vi "CT_CapVoltCamBinning.vi"(2 "Bin Size Reduction":i32, 3 "Center Spacing Y":dbl, 4 "Center Spacing X":dbl, 5 "Boundry Pixel Array":T1(array[cluster])=[{"Location Label"="Top  Left", "X Pixel"=0, "Y pixel"=0}, {"Location Label"="Top Right", "X Pixel"=0, "Y pixel"=0}, {"Location Label"="Bottom Right", "X Pixel"=0, "Y pixel"=0}, {"Location Label"="Bottom Left", "X Pixel"=0, "Y pixel"=0}]) -> (0 "Bin Center Array":cluster{"X":i32, "Y":i32}[][](array[cluster]), 1 "Fiber Bin Array":u32[][](array[numeric]))   [LabVIEW 2016]
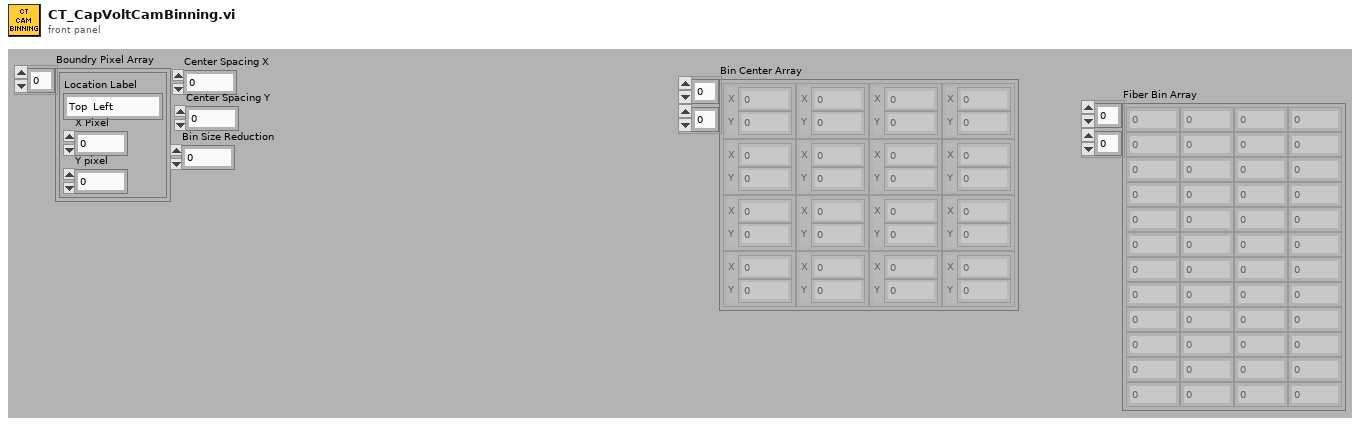
[diagram p1: front panel]
types:
  T1 = cluster{"Location Label":string, "X Pixel":i32, "Y pixel":i32}[]
  T2 = cluster{"Location Label":string, "X Pixel":i32, "Y pixel":i32}
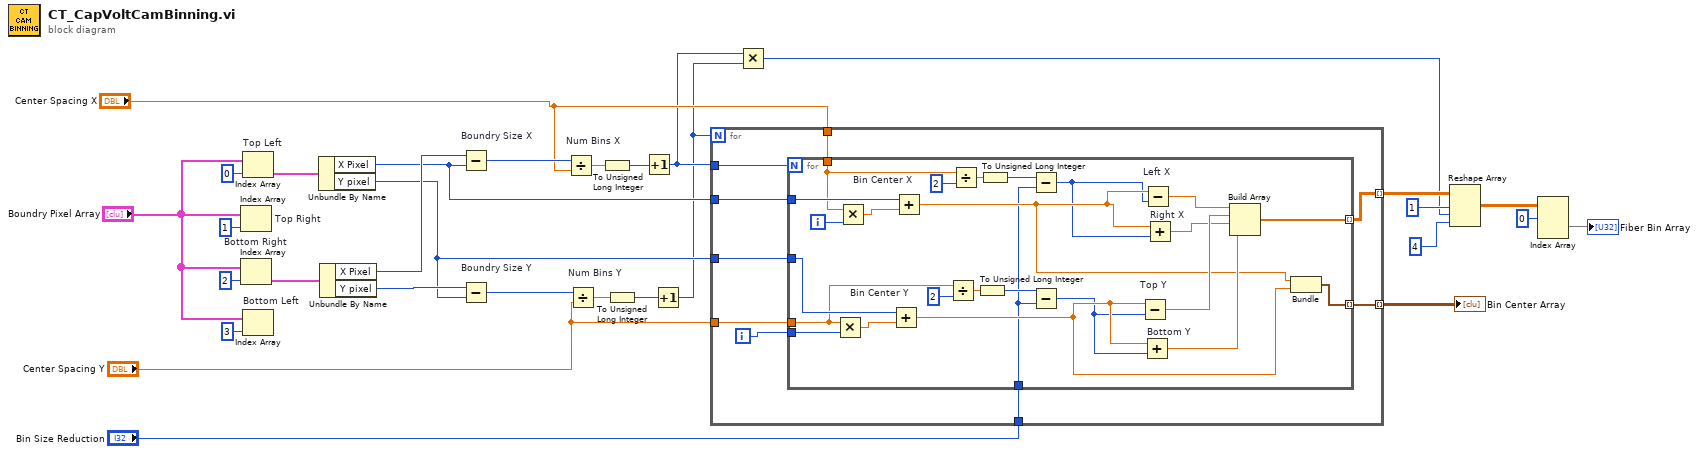
[diagram p0: block diagram]
diagram:
  n1 = Index Array "Top Right"(array="Boundry Pixel Array", index=1) -> ()  [unwired: 1 out]
  n2 = Index Array "Bottom Right"(array="Boundry Pixel Array", index=2) -> (element=w24:T2)
  n3 = Index Array "Top Left"(array="Boundry Pixel Array", index=0) -> (element=w25:T2)
  n4 = Index Array "Bottom Left"(array="Boundry Pixel Array", index=3) -> ()  [unwired: 1 out]
  n5 = Unbundle By Name(w25) -> ("X Pixel"=w17:i32, "Y pixel"=w15:i32)
  n6 = Unbundle By Name(w24) -> ("X Pixel"=w23:i32, "Y pixel"=w22:i32)
  n7 = Subtract "Boundry Size X"(x=w23, y=w17) -> (x-y=w21:i32)
  n8 = Subtract "Boundry Size Y"(x=w22, y=w15) -> (x-y=w20:i32)
  n9 = Divide "Num Bins X"(x=w21, y="Center Spacing X") -> (x/y=w19:dbl)
  n10 = Divide "Num Bins Y"(x=w20, y="Center Spacing Y") -> (x/y=w18:dbl)
  n11 = To Unsigned Long Integer(number=w19) -> (unsigned 32bit integer=w12:u32)
  n12 = To Unsigned Long Integer(number=w18) -> (unsigned 32bit integer=w11:u32)
  n13 = Increment(x=w12) -> (x+1=w7:u32)
  n14 = Increment(x=w11) -> (x+1=w6:u32)
  n15 = for {
    N: w6 -> [_]
    tunnel: w7 -> [w39]
    tunnel: w17 -> [w38]
    tunnel: "Center Spacing X" -> [w37]
    tunnel: w15 -> [w36]
    tunnel: "Center Spacing Y" -> [w35]
    tunnel: [w33] -> w13 mode=indexing
    tunnel: [w32] -> w10 mode=indexing
    tunnel: "Bin Size Reduction" -> [w31]
    i -> [w34]
    n16 = for {
      N: w39 -> [_]
      tunnel: w38 -> [w64]
      tunnel: w37 -> [w61]
      tunnel: w36 -> [w54]
      tunnel: w34 -> [w55]
      tunnel: w35 -> [w53]
      tunnel: [w48] -> w32 mode=indexing
      tunnel: [w47] -> w33 mode=indexing
      tunnel: w31 -> [w40]
      i -> [w63]
      n17 = Multiply(x=w53, y=w55) -> (x*y=w58:dbl)
      n18 = Multiply(x=w61, y=w63) -> (x*y=w62:dbl)
      n19 = Add "Bin Center Y"(x=w54, y=w58) -> (x+y=w45:dbl)
      n20 = Add "Bin Center X"(x=w64, y=w62) -> (x+y=w46:dbl)
      n21 = Divide(x=w53, y=2) -> (x/y=w56:dbl)
      n22 = Divide(x=w61, y=2) -> (x/y=w59:dbl)
      n23 = To Unsigned Long Integer(number=w56) -> (unsigned 32bit integer=w44:u32)
      n24 = To Unsigned Long Integer(number=w59) -> (unsigned 32bit integer=w42:u32)
      n25 = Subtract(x=w42, y=w40) -> (x-y=w41:u32)
      n26 = Subtract(x=w44, y=w40) -> (x-y=w43:u32)
      n27 = Subtract "Top Y"(x=w45, y=w43) -> (x-y=w51:dbl)
      n28 = Add "Bottom Y"(x=w45, y=w43) -> (x+y=w49:dbl)
      n29 = Subtract "Left X"(x=w46, y=w41) -> (x-y=w52:dbl)
      n30 = Add "Right X"(x=w46, y=w41) -> (x+y=w50:dbl)
      n31 = Build Array(w52, w51, w50, w49) -> (w48:dbl[])
      n32 = Bundle(w46, w45) -> (w47:cluster{dbl, dbl})  [unwired: 1 in]
    }
  }
  "Bin Center Array" <- w13
  n33 = Multiply(x=w7, y=w6) -> (x*y=w5:u32)
  n34 = Reshape Array(w10, 1 ("dimension size"), w5, 4 ("dimension size")) -> (w4:dbl[][][])
  n35 = Index Array(array=w4, index (dim 0)=0 ("index (page)")) -> (element=→"Fiber Bin Array":dbl[][])  [unwired: 2 in]
